vi "Write Section - Array (String).vi"(6 "Create file if not found? (T)":bool=TRUE, 7 "Value":string[](array[string]), 8 "error in (no error)":errorcluster, 9 "key":string, 10 "section":string, 11 "Path":path) -> (0 "error out":errorcluster)   [LabVIEW 2019, in "TSC File IO.lvlib"]
doc: "This VI will write a section/key configuration file of the type:\n<b>array of strings</b>\n\nInputs:\n-Path [path] - a path to the file\n-section [string] - the section string in the configuration file\n-key [string] - the key to be read in the configuration file\n-value [array of String] - the output data written\n-error in\n\nOutputs:\n-error out\n\n<b>Code Developed By:</b>\nDaniel Coons\nTechnology Service Corporation\n1983 S Liberty Drive\nBloomington, IN 47403\nwww.tsc.com\\atcs"
uses:
  TSC File IO.lvlib
  <vilib>/Utility/config.llb/Write Key (String).vi
  <vilib>/Utility/config.llb/NI_LVConfig.lvlib
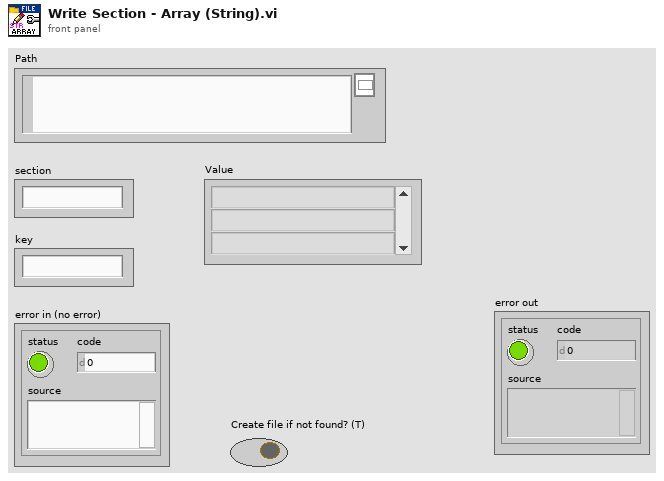
[diagram p1: front panel]
types:
  T1 = typedef "NI_LVConfig.lvlib/Config Data RefNum.ctl" = refnum<k1>
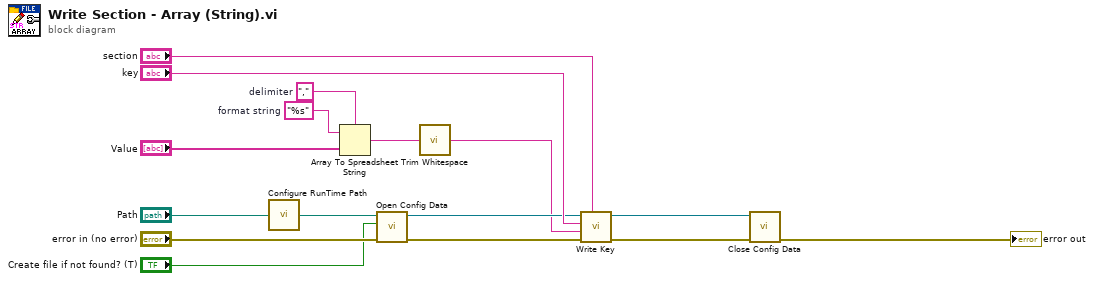
[diagram p0: block diagram]
diagram:
  w8 = "%s"  # format string
  w9 = ","  # delimiter
  n1 = call "Configure RunTime Path.vi"("Input Path"="Path") -> ("Updated Path"=w6:path)
  n2 = Array To Spreadsheet String(delimiter (Tab)=w9, array="Value", 3:w8) -> (spreadsheet string=w2:string)
  n3 = call <vilib>:"Open Config Data.vi"("error in (no error)"="error in (no error)", "create file if necessary (T)"="Create file if not found? (T)", "configuration file path"=w6) -> ("error out"=w10:errorcluster, "refnum"=w11:T1)  [unwired: 6 in, 1 out]
  n4 = call <vilib>:"Trim Whitespace.vi"("string"=w2) -> ("trimmed string"=w1:string)  [unwired: 1 in]
  n5 = call-poly <vilib>:"Write Key.vi"("section"="section", "error in (no error)"=w10, "value"=w1, "key"="key", "refnum"=w11) -> ("error out"=w7:errorcluster, "refnum out"=w12:T1)  [unwired: 4 in, 1 out]
  n6 = call <vilib>:"Close Config Data.vi"("error in (no error)"=w7, "refnum"=w12) -> ("error out"=→"error out":errorcluster)  [unwired: 8 in, 1 out]
